vi "Is In Place Bundler.vi"(10 "User VI Ref":refnum<vi>, 11 "Affected Items":T1) -> (0 "Terminal Ct":i32, 1 "First Term Selected":bool, 3 "In Place Bundler Selected":bool, 4 "Data Type":variant)   [LabVIEW 2023]
doc: "Determine if selected BD terminals are In-place bundler nodes and whether the first item is selected."
uses:
  top/BundleMagic.ctl
  <vilib>/Utility/Data Type/NI_Data Type.lvlib
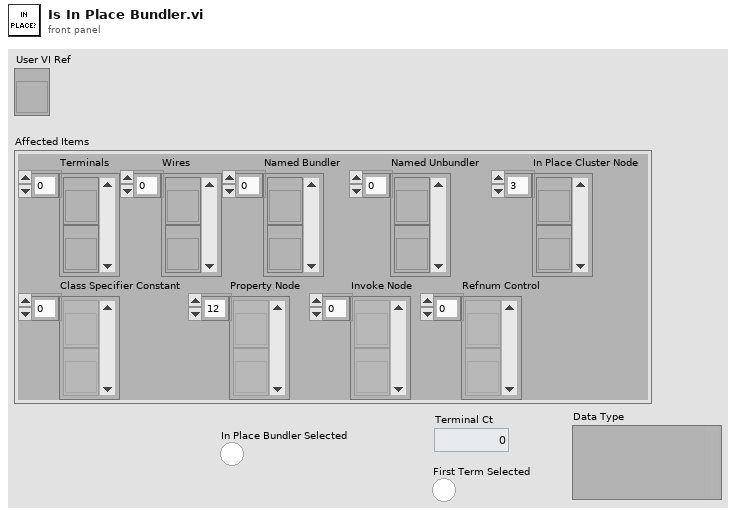
[diagram p1: front panel]
types:
  T1 = typedef "BundleMagic.ctl" = cluster{"Terminals":refnum<vi>[], "Wires":refnum<vi>[], "Named Bundler":refnum<vi>[], "Named Unbundler":refnum<vi>[], "In Place Cluster Node":refnum<vi>[], "Class Specifier Constant":refnum<vi>[], "Property Node":refnum<vi>[], "Invoke Node":refnum<vi>[], "Refnum Control":refnum<vi>[]}
  T2 = typedef "NI_Data Type.lvlib/Data Type.ctl" = enum8{"Invalid Type", "Void", "I8", "I16", "I32", "I64", "U8", "U16", "U32", "U64", "Single Float", "Double Float", "Extended Float", "Single Complex", "Double Complex", "Extended Complex", "Enum U8", "Enum U16", "Enum U32", "Enum U64", "Single Float With Unit", "Double Float With Unit", "Extended Float With Unit", "Single Complex with Unit", "Double Complex with Unit", "Extended Complex with Unit", "Boolean", "String", "Path", "Picture", "Tag", "Array", "Cluster", "Variant", "LV Variant", "Waveform", "Timestamp", "Digital Waveform", "Digital Data", "ExpressData", "Refnum", "External Data", "VI", "Poly VI", "LabVIEW Class Instance", "Fixed Point", "Set Collection", "Map Collection"}
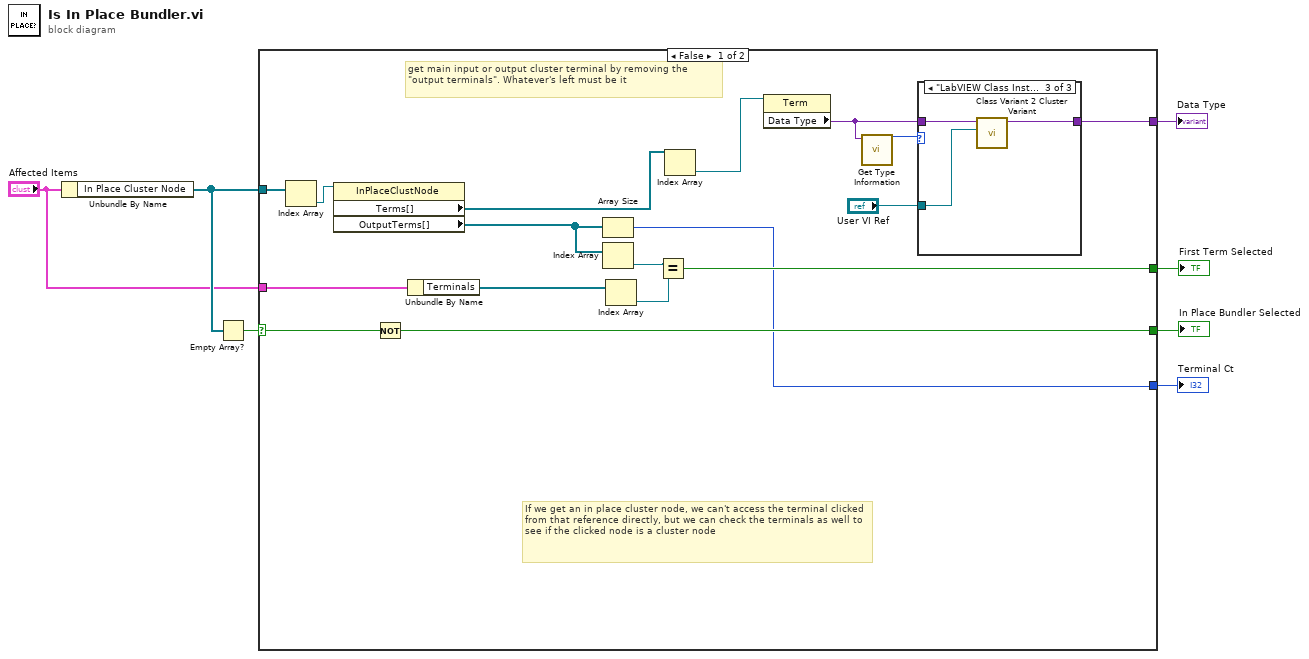
[diagram p0: block diagram]
diagram:
  n1 = Unbundle By Name("Affected Items") -> ("In Place Cluster Node"=w7:refnum<vi>[])
  n2 = Empty Array?(array=w7) -> (empty?=w5:bool)
  n3 = case shown="False" w5 {
    selector: w5 -> [w14 _]
    tunnel: w7 -> [w24 _]
    tunnel: "Affected Items" -> [w22 _]
    tunnel: [w11 _] -> w4
    tunnel: [w10 _] -> w3
    tunnel: [w9 _] -> w2
    tunnel: [w8 _] -> w1
    frame False {
      # "get main input or output cluster terminal by removing the \"output terminals\". Whatever's left must be it"
      # "If we get an in place cluster node, we can't access the terminal clicked from that reference directly, but we can check the terminals as well to see if the clicked node is a cluster node"
      n4 = Index Array(array=w24) -> (element=w23:refnum<vi>)  [unwired: 1 in]
      n5 = property class="InPlaceClustNode"(reference=w23) -> ("Terms[]"=w12:refnum<vi>[], "OutputTerms[]"=w13:refnum<vi>[])  [unwired: 1 in, 2 out]
      n6 = Not(x=w14) -> (.not. x?=w10:bool)
      n7 = Unbundle By Name(w22) -> ("Terminals"=w21:refnum<vi>[])
      n8 = Array Size(array=w13) -> (size(s)=w8:i32)
      n9 = Index Array(array=w13) -> (element=w20:refnum<vi>)  [unwired: 1 in]
      n10 = Index Array(array=w21) -> (element=w19:refnum<vi>)  [unwired: 1 in]
      n11 = Equal?(x=w20, y=w19) -> (x = y?=w9:bool)
      n12 = Index Array(array=w12) -> (element=w18:refnum<vi>)  [unwired: 1 in]
      n13 = property class="Term"(reference=w18) -> ("Data Type"=w15:variant)  [unwired: 1 in, 2 out]
      n14 = call <vilib>:"Get Type Information.vi"("variant"=w15) -> ("type"=w17:T2)  [unwired: 6 in, 4 out]
      n15 = case shown="\"LabVIEW Class Instance\"" w17 {
        tunnel: w15 -> [w25 w26 w29]
        tunnel: [w25 w26 w28] -> w11
        tunnel: "User VI Ref" -> [_ _ w27]
        frame "Invalid Type", Default {
        }
        frame "Cluster" {
        }
        frame "LabVIEW Class Instance" {
          n16 = call "Class Variant 2 Cluster Variant.vi"("User VI Ref"=w27, "Variant"=w29) -> ("Control Value:Get"=w28:variant)  [unwired: 8 in, 1 out]
        }
      }
    }
    frame True {
    }
  }
  "Data Type" <- w4
  "First Term Selected" <- w2
  "In Place Bundler Selected" <- w3
  "Terminal Ct" <- w1
